vi "Filter.vi"(4 "Clip units of Ts off":dbl, 6 "Fix time delay":bool=TRUE, 7 "Filter type":enum16{"None", "IIR", "FIR"}(ring), 8 "Error In":errorcluster, 10 "Time constant":dbl=0.0001 format="%#_6p", 11 "Data":waveform(dbl)[](array[waveform])) -> (0 "Error Out":errorcluster, 2 "Settings":string, 3 "Data out":waveform(dbl)[](array[waveform]))   [LabVIEW 2015]
uses:
  IIR Filter parameters.ctl
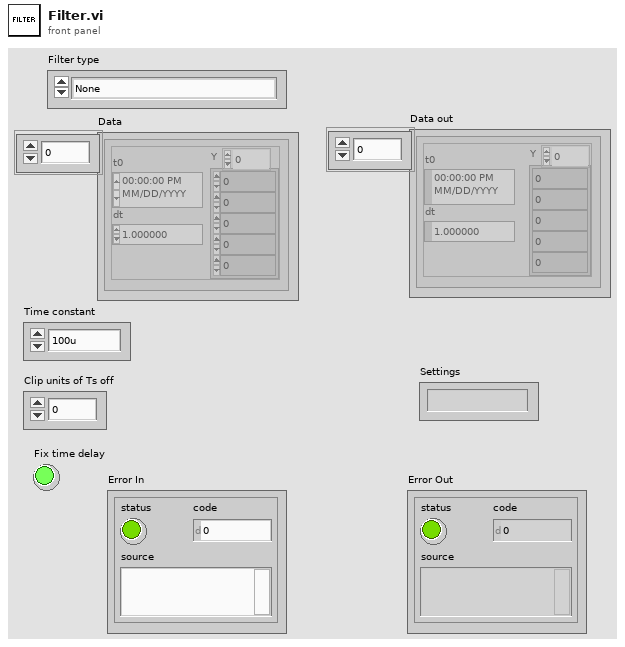
[diagram p1: front panel]
types:
  T1 = typedef "IIR Filter parameters.ctl" = cluster{"Clip off ramp-up, 1/Fc":dbl, "Double-pass in reverse":bool, "IIR filter specifications":cluster{"Topology":enum16{"Off", "Butterworth", "Chebyshev", "Inverse Chebyshev", "Elliptic", "Bessel"}, "Type":enum16{"Lowpass", "Highpass", "Bandpass", "Bandstop"}, "Order":i32, "Lower Fc":dbl, "Upper Fc":dbl, "PB Ripple":dbl, "SB Attenuation":dbl}}
  T2 = cluster{"Clip IIR filter ramps, 1/Fc":dbl, "Two-pass & flip":bool, "FIR filter specifications":cluster{"Topology":enum16{"Off", "FIR by Specification", "Equi-ripple FIR", "Windowed FIR"}, "Type":enum16{"Lowpass", "Highpass", "Bandpass", "Bandstop"}, "#Taps":i32, "Lower PB":dbl, "Upper PB":dbl, "Lower SB":dbl, "Upper SB":dbl}, "optional FIR filter\n specifications":cluster{"PB Gain":dbl, "SB Gain":dbl, "Scale":bool, "Window":enum16{"None", "Hanning", "Hamming", "Triangular", "Blackman", "Exact Blackman", "Blackman-Harris", "Kaiser-Bessel", "Flat Top"}}}
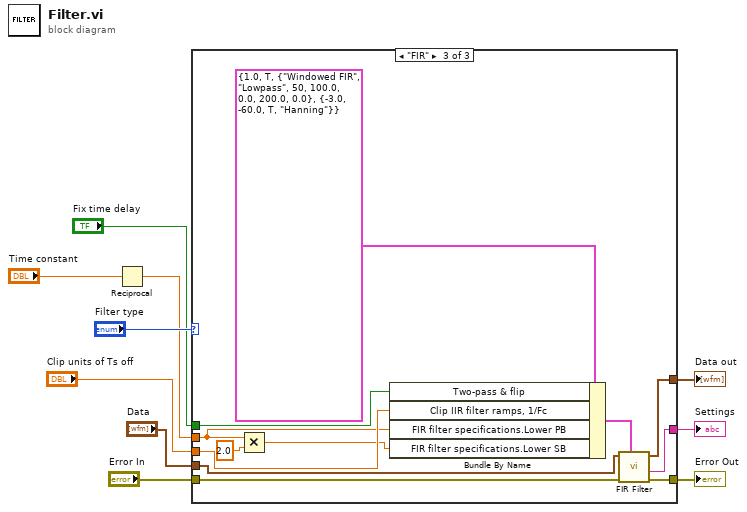
[diagram p0: block diagram]
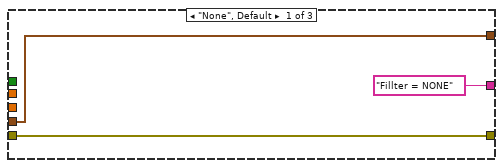
[diagram p2: hidden frame]
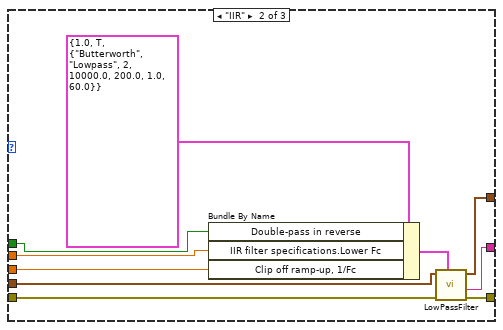
[diagram p3: hidden frame]
diagram:
  n1 = Reciprocal(x="Time constant") -> (1/x=w4:dbl)
  n2 = case shown="\"FIR\"" "Filter type" {
    tunnel: "Data" -> [w13 w23 w34]
    tunnel: [w13 w17 w33] -> w8
    tunnel: "Error In" -> [w12 w22 w35]
    tunnel: "Fix time delay" -> [_ w19 w27]
    tunnel: w4 -> [_ w18 w26]
    tunnel: [w12 w16 w32] -> w3
    tunnel: "Clip units of Ts off" -> [_ w15 w28]
    tunnel: ["Fillter = NONE" ("Settings out") w14 w31] -> w1
    frame "None", Default {
    }
    frame "IIR" {
      n3 = Bundle By Name(cluster=T1 {"Clip off ramp-up, 1/Fc"=1.0, "Double-pass in reverse"=TRUE, "IIR filter specifications"={"Topology"=enum."Butterworth", "Type"=enum."Lowpass", "Order"=2, "Lower Fc"=10000.0, "Upper Fc"=200.0, "PB Ripple"=1.0, "SB Attenuation"=60.0}} ("Low-pass filter"), "Double-pass in reverse"=w19, "IIR filter specifications.Lower Fc"=w18, "Clip off ramp-up, 1/Fc"=w15) -> (w20:T1)
      n4 = call "LowPassFilter.vi"("Low-pass filter"=w20, "error in (no error)"=w22, "signal(s) in"=w23) -> ("error out"=w16:errorcluster, "Settings out"=w14:string, "signal(s) out"=w17:waveform(dbl)[])  [unwired: 5 in, 1 out]
    }
    frame "FIR" {
      n5 = Multiply(x=w26, y=2.0) -> (x*y=w24:dbl)
      n6 = Bundle By Name(cluster=T2 {"Clip IIR filter ramps, 1/Fc"=1.0, "Two-pass & flip"=TRUE, "FIR filter specifications"={"Topology"=enum."Windowed FIR", "Type"=enum."Lowpass", "#Taps"=50, "Lower PB"=100.0, "Upper PB"=0.0, "Lower SB"=200.0, "Upper SB"=0.0}, "optional FIR filter\n specifications"={"PB Gain"=-3.0, "SB Gain"=-60.0, "Scale"=TRUE, "Window"=enum."Hanning"}} ("FIR Low-pass filter"), "Two-pass & flip"=w27, "Clip IIR filter ramps, 1/Fc"=w28, "FIR filter specifications.Lower PB"=w26, "FIR filter specifications.Lower SB"=w24) -> (w29:T2)
      n7 = call "FIR Filter.vi"("FIR Low-pass filter"=w29, "error in (no error)"=w35, "signal(s) in"=w34) -> ("error out"=w32:errorcluster, "Settings out"=w31:string, "signal(s) out"=w33:waveform(dbl)[])  [unwired: 5 in, 1 out]
    }
  }
  "Data out" <- w8
  "Error Out" <- w3
  "Settings" <- w1
